vi "eSerial_Protekkkk.vi"(2 "string to write":string="*IDN?", 3 "VISA resource name (write)":refnum<visa-resource-name>="COM4") -> (0 "error out":errorcluster, 1 "read string":string)   [LabVIEW 2011]
doc: "The Advanced Serial Read and Write example performs a Serial Port Read, a Serial Port Write, or a combination of these actions while setting some advanced serial features like buffer size, termination characters, and XON/XOFF flow control. The user selects the actions (read or write) on the front panel. If both are selected, the VI will write the data first, read the data and then close the VISA session that is opened to the port. \n\nThe parameters set for the serial port must match the parameters of the connected instrument or device. In this example, the bytes to read parameter specifies the number of bytes that the serial port reads. If there were more bytes at the port than the number specified in bytes to read, those bytes would not be read. Also, if you specify to read more bytes than the number of bytes actually read, you might receive a timeout error message.\n\nINSTRUCTIONS:\n1) Select the serial resource and configuration parameters (baud rate, data bits, parity, stop bits, flow control).\n2) Termination character can be enabled and set. Also, set the required input buffer size prior to running the example.\n3) Select the operations to be performed. \n4) Connect the serial port to your device. If no device is available, perform a loopback test by doing one of the following. Short pins 2 and 3 on a RS-232 cable or short pin 4 to pin 8 and pin 5 to pin 9 on a RS-485/422 cable. \n5) Run the VI to see the data read. (The \"read string\" will match the \"string to write\" if a loopback test was performed.)\n\nThis example exposes several advanced features that you may need for your application. Not all applications need all the features shown in this example. The input buffer size is likely an important setting that you want to control in your application. This example expands upon the flow control option for XON and XOFF, allowing the user to choose those control characters. The timeout parameter has been brought to the front panel so a user can specify the time period the VISA Read will wait for the number of bytes to read before timing out. Also, the user has several controls for the termination character, which is discussed later.\n\nNote that you can press the write and read buttons and change the bytes to read parameters on the fly, while the example is running. However, you must stop the example to change the other configuration parameters after the example has started running, and then run again.\n\nSet the I/O buffer size slightly higher the amount of data you expect to receive. This is very important for applications that don't use flow control, as you may lose characters if the receive buffer overflows.\n\nSetting the timeout period ensures that the operation returns with a timeout error if the operation cannot be performed in the specified time period. \n\nSome devices require a termination character in order to identify the end of command strings. Some devices send a termination character to signify the end of data to be read. \n\nThis example shows how you can end the Read operation once a termination character is detected in the buffer and/or append a termination character at the end of the Write data. To enable the Read to end on a termination character, use the VISA Configure Serial Port or use the VISA Properties Serial End Mode for Reads, Termination Character Enable, and Termination Character. To end the Write with a termination character, use the VISA Properties Serial End Mode for Writes, the Send End Enable, and Termination Character. In this example, the same termination character is used for both the Read and the Write. You can specify two different characters for your application, if desired.\n\nYour application may require specific characters for the XON/XOFF Flow Control. You can specify these characters with the VISA Properties Flow Control XOFF Character and Flow Control XON Character. Note that if the standard XON and XOFF characters are used, then decimal 17 and 19 are unavailable for data values. Remember that using flow control and setting an adequate buffer size allow you to prevent buffer overflows."
uses:
  <vilib>/Instr/_visa.llb/VISA Configure Serial Port (Instr).vi
panel:
  out "x-y 3":u32
  out "x-y 2":u32
  out "x-y":u32
  in  "baud rate (9600)":u32=9600
  in  "data bits (8)":u16=8 min=5 max=8 step=1
  in  "parity (0:none)":u16(ring) items=["None", "Odd", "Even", "Mark", "Space"]
  in  "flow control":u16(ring) items=["None"=0, "XON/XOFF"=1, "RTS/CTS"=2, "DTR/DSR"=4]
  in  "stop bits":u16(ring)=10 items=["1.0"=10, "1.5"=15, "2.0"=20]
  in  "Port Sec 2":refnum<visa-resource-name>="COM1"
  in  "Port Sec":refnum<visa-resource-name>="COM1"
  out "bytes written":u32
  out "actual bytes read":u32
  # "On Windows/Linux, consider using the Instrument Driver Finder (Help>>Find Instrument Drivers) to search for an instrument driver for your instrument."
  # "Select the serial resource and the operations to be performed.  If all are selected, the VI will write the data first, read data and then close the VISA session that is opened to the port.  This VI will wait until the specified number of bytes is received at the port, until the timeout period is met, or until a termination character is received.  The default termination character in this example is the Line Feed ( ASCII 0xA, '\\n' ).  Also, set the required input buffer size prior to running the example.\nNote: The example loops until the STOP button is pressed."
  # "For additional information select File >> VI Properties >> Documentation"
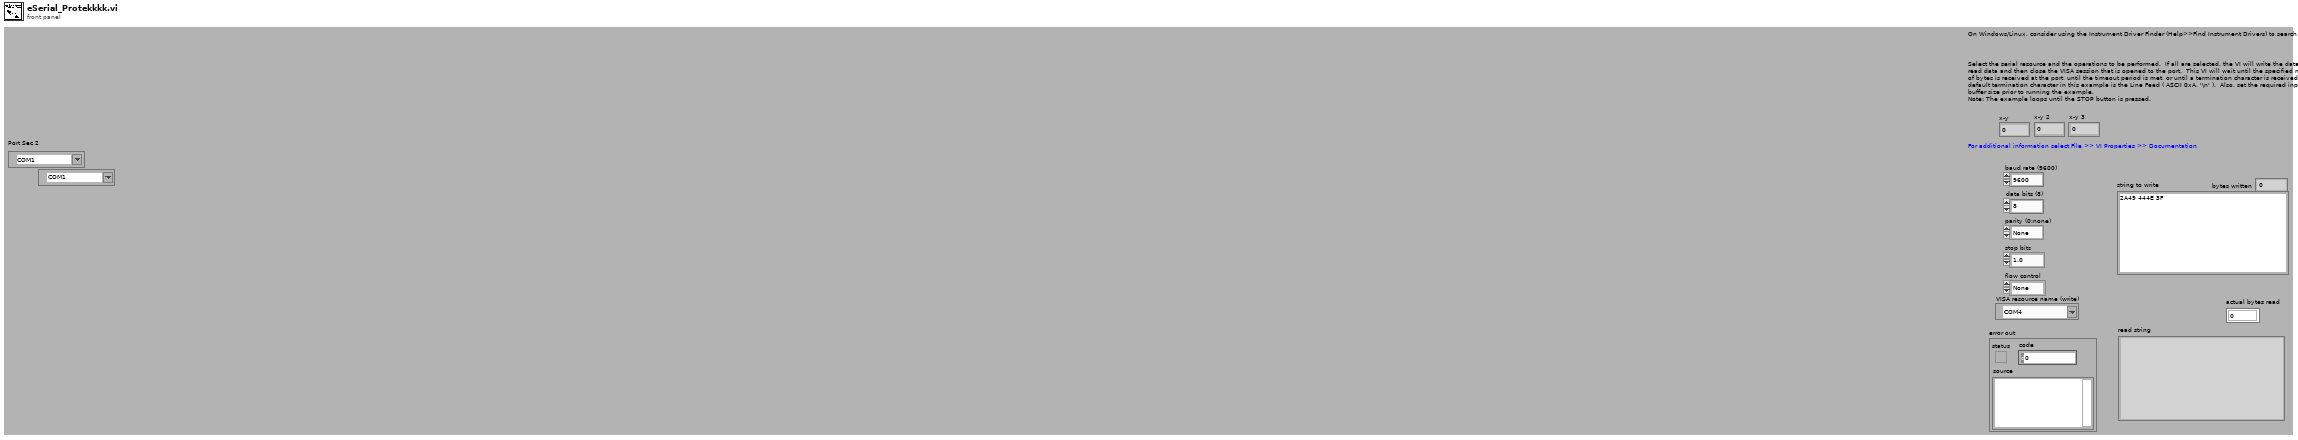
[diagram p1: front panel]
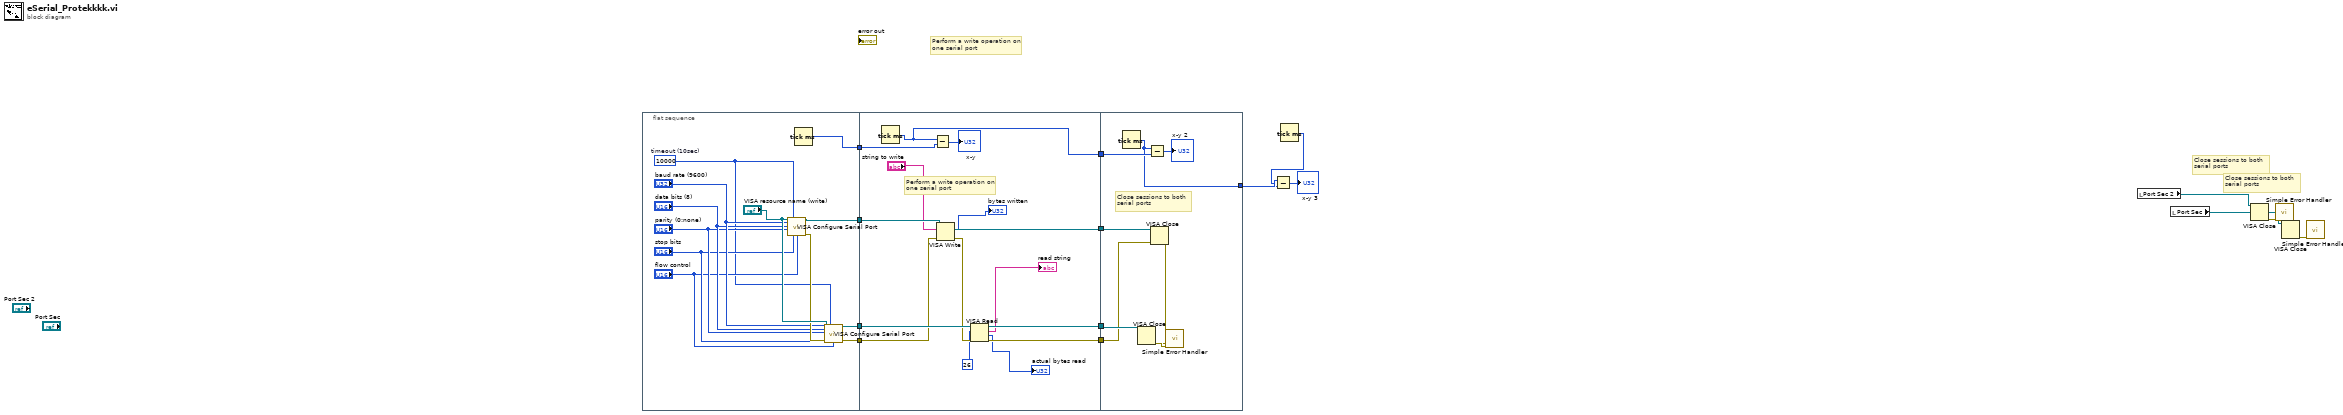
[diagram p0: block diagram]
diagram:
  # "Close sessions to both serial ports"
  # "Close sessions to both serial ports"
  # "Perform a write operation on one serial port"
  n1 = flat-sequence {
    tunnel: [w19] -> w11
    tunnel: [w18] -> w10
    tunnel: [w17] -> w9
    tunnel: [w16] -> w8
    tunnel: w11 -> [w42]
    tunnel: w10 -> [w41]
    tunnel: w9 -> [w40]
    tunnel: [w38] -> w7
    tunnel: [w37] -> w6
    tunnel: [w36] -> w5
    tunnel: w8 -> [w34]
    tunnel: [w32] -> w4
    tunnel: w7 -> [w47]
    tunnel: w6 -> [w46]
    tunnel: w5 -> [w48]
    tunnel: w4 -> [w45]
    tunnel: [w43] -> w2
    frame #0 {
      w20 = u32 10000  # timeout (10sec)
      n2 = call-poly "VISA Configure Serial Port"("VISA resource name"="VISA resource name (write)", "timeout (10sec)"=w20, "baud rate (9600)"="baud rate (9600)", "data bits (8)"="data bits (8)", "parity (0:none)"="parity (0:none)", "stop bits (10: 1 bit)"="stop bits", "flow control (0:none)"="flow control") -> ("VISA resource name out"=w19:refnum<visa-resource-name>, "error out"=w26:errorcluster)  [unwired: 2 in, 5 out]
      n3 = Tick Count (ms)() -> (millisecond timer value=w16:u32)
      n4 = call-poly "VISA Configure Serial Port"("VISA resource name"="VISA resource name (write)", "timeout (10sec)"=w20, "baud rate (9600)"="baud rate (9600)", "data bits (8)"="data bits (8)", "parity (0:none)"="parity (0:none)", "error in (no error)"=w26, "stop bits (10: 1 bit)"="stop bits", "flow control (0:none)"="flow control") -> ("VISA resource name out"=w18:refnum<visa-resource-name>, "error out"=w17:errorcluster)  [unwired: 2 in, 4 out]
    }
    frame #1 {
      # "Perform a write operation on one serial port"
      n5 = Tick Count (ms)() -> (millisecond timer value=w32:u32)
      n6 = Subtract(x=w32, y=w34) -> (x-y=→"x-y":u32)
      n7 = VISA Write(VISA resource name=w42, write buffer="string to write", error in (no error)=w40) -> (VISA resource name out=w36:refnum<visa-resource-name>, return count=→"bytes written":u32, error out=w39:errorcluster)
      n8 = VISA Read(VISA resource name=w41, byte count=u32 26, error in (no error)=w39) -> (VISA resource name out=w38:refnum<visa-resource-name>, read buffer=→"read string":string, return count=→"actual bytes read":u32, error out=w37:errorcluster)
    }
    frame #2 {
      # "Close sessions to both serial ports"
      n9 = Tick Count (ms)() -> (millisecond timer value=w43:u32)
      n10 = Subtract(x=w43, y=w45) -> (x-y=→"x-y 2":u32)
      n11 = VISA Close(VISA resource name=w48, error in (no error)=w46) -> (error out=w49:errorcluster)
      n12 = VISA Close(VISA resource name=w47, error in (no error)=w49) -> (error out=w50:errorcluster)
      n13 = call <vilib>:"Simple Error Handler.vi"("error in (no error)"=w50) -> ()  [unwired: 1 in, 8 out]
    }
  }
  n14 = Tick Count (ms)() -> (millisecond timer value=w1:u32)
  n15 = Subtract(x=w2, y=w1) -> (x-y=→"x-y 3":u32)
  n16 = local read "Port Sec 2"() -> (w13:refnum<visa-resource-name>)
  n17 = local read "Port Sec"() -> (w15:refnum<visa-resource-name>)
  n18 = VISA Close(VISA resource name=w13) -> (error out=w12:errorcluster)  [unwired: 1 in]
  n19 = call <vilib>:"Simple Error Handler.vi"("error in (no error)"=w12) -> ()  [unwired: 1 in, 8 out]
  n20 = VISA Close(VISA resource name=w15) -> (error out=w14:errorcluster)  [unwired: 1 in]
  n21 = call <vilib>:"Simple Error Handler.vi"("error in (no error)"=w14) -> ()  [unwired: 1 in, 8 out]
